vi "Apply.vi"(8 "error in (no error)":errorcluster, 11 "NEO480HTA Base CFG in":refnum<class "Read All CFG.lvclass">) -> (0 "error out":errorcluster, 3 "NEO480HTA Base CFG out":refnum<class "Read All CFG.lvclass">)   [LabVIEW 2023, in "NEO480HTA.lvlib" / "Read All CFG.lvclass"]
uses:
  Read All CFG.lvclass
  D:/git/HAL/HAL GOOP4/Configuration JSON Base/CFG JSON Base.lvclass
  Configuration JSON Base/CFG JSON Base.lvclass/CFG JSON Base.ctl
  Read All CFG.lvclass/Read All CFG.ctl
  9bca5c5c-edef-47c5-918c-bf756a254fce.vi
  fc27cf02-12b1-46f5-bd0d-6de24ae4e0a7.vi
  bc72a19a-b621-4a94-833b-c6b45453ec49.vi
  0be9cb3e-7191-46de-b2d2-d721f6475833.vi
  <vilib>/JDP Science/JSONtext/Find Item.vi
  <vilib>/JDP Science/JSONtext/Next JSON Value.vi
  <vilib>/JDP Science/JSONtext/String Subset.vi
  <vilib>/JDP Science/JSONtext/Parsing/Advance past next JSON Value (inlined COPY).vi
  <vilib>/JDP Science/JSONtext/Parsing/Advance past whitespace.vi
  <vilib>/JDP Science/JSONtext/Parsing/Advance past String.vi
  <vilib>/JDP Science/JSONtext/Parsing/Advance past Number.vi
  <vilib>/JDP Science/JSONtext/Parsing/Advance past Line Ending.vi
  <vilib>/JDP Science/JSONtext/Parsing/Parse Full Path or Item Name.vi
  <vilib>/JDP Science/JSONtext/Parsing/Advance past Array.vi
  <vilib>/JDP Science/JSONtext/Parsing/Advance past Object.vi
  <vilib>/JDP Science/JSONtext/support/Error Cluster From Code.vi
  <vilib>/JDP Science/JSONtext/Offset/Find Item Locations by Path.vi
  <vilib>/JDP Science/JSONtext/JSON text to Variant.vi
  <vilib>/Utility/error.llb/Error Cluster From Error Code.vi
  <vilib>/xnet/xnet.llb/XNET Create Session (Frame Input Single-point).vi
  <vilib>/JDP Science/JSONtext/LVClass Serializer/JSONtext LVClass Serializer.lvclass
  <vilib>/ErrorRing/Error Ring.xnode
  Configuration JSON Base/CFG JSON Base.lvclass
  <resource>/objmgr/xnet.rc
panel:
  out "Interface:CAN:Termination":u32(ring)=1 items=["Off", "On"]
  out "Timing Type":u32(ring)=1 items=["Cyclic Data", "Event Data", "Cyclic Remote", "Event Remote"]
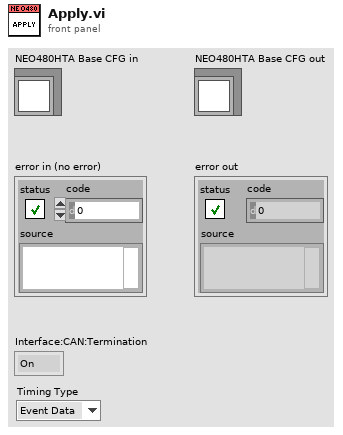
[diagram p1: front panel]
types:
  T1 = cluster{"Baud Rate":u32, "Comment":string, "Name":string}
  T2 = cluster{"Frame name":string, "Identifier":u32, "Payload Length":u32, "Timing Type":string, "Transmit Time":dbl, "Extended Identifier?":bool, "Comment":string}[]
  T3 = cluster{"Frame name":string, "Identifier":u32, "Payload Length":u32, "Timing Type":u32, "Transmit Time":dbl, "Extended Identifier?":bool, "Comment":string}
  T4 = typedef "LVStringsAndValuesArrayTypeDef_U32.ctl" = cluster{"String":string, "Value":u32}[]
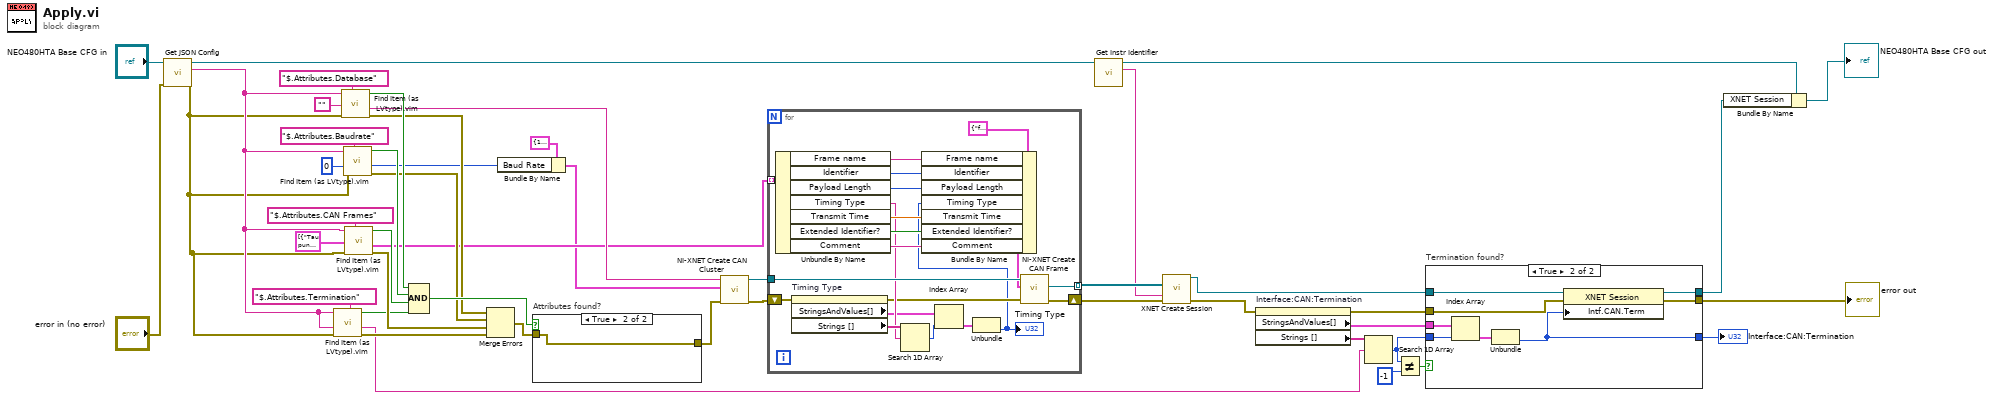
[diagram p0: block diagram]
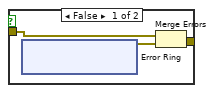
[diagram p3: hidden frame]
diagram:
  n1 = call "Get JSON Config.vi"("error in (no error)"="error in (no error)", "CFG Base in"="NEO480HTA Base CFG in") -> ("error out"=w7:errorcluster, "<JSON>Config>"=w8:string, "CFG Base out"=w29:refnum<class "Read All CFG.lvclass">)  [unwired: 7 in]
  n2 = call "Find Item (as LVtype).vim"("$Path or Item Name"="$.Attributes.Termination", "error in (no error)"=w7, "Data Type and Default Value"=w8, "JSON"=w8) -> ("error out"=w26:errorcluster, "Data"=w12:string, "Found"=w27:bool)  [unwired: 4 in, 1 out]
  n3 = call "Find Item (as LVtype).vim"("$Path or Item Name"="$.Attributes.Database", "error in (no error)"=w7, "Data Type and Default Value"="", "JSON"=w8) -> ("error out"=w33:errorcluster, "Data"=w40:string, "Found"=w41:bool)  [unwired: 4 in, 1 out]
  n4 = call "Find Item (as LVtype).vim"("$Path or Item Name"="$.Attributes.Baudrate", "error in (no error)"=w7, "Data Type and Default Value"=u32 0, "JSON"=w8) -> ("error out"=w34:errorcluster, "Data"=w20:u32, "Found"=w44:bool)  [unwired: 4 in, 1 out]
  n5 = call "Find Item (as LVtype).vim"("$Path or Item Name"="$.Attributes.CAN Frames", "error in (no error)"=w7, "Data Type and Default Value"=T2 [{"Frame name"="Taupunkt", "Identifier"=1152, "Payload Length"=8, "Timing Type"="Event Data", "Transmit Time"=0.0, "Extended Identifier?"=FALSE, "Comment"=""}], "JSON"=w8) -> ("error out"=w35:errorcluster, "Data"=w17:T2, "Found"=w45:bool)  [unwired: 4 in, 1 out]
  n6 = Compound Arithmetic op=AND(w41, w44, w45, w27) -> (w43:bool)
  n7 = Merge Errors(w33, w34, w35, w26) -> (w36:errorcluster)
  n8 = Bundle By Name(cluster=T1 {"Baud Rate"=125000, "Comment"="", "Name"="x"} ("CAN Cluster"), "Baud Rate"=w20) -> (w1:T1)
  n9 = case "Attributes found?" shown="True" w43 {
    tunnel: w36 -> [w49 w56]
    tunnel: [w50 w56] -> w39
    frame False {
      n10 = xnode "Error Ring"() -> ("error out"=w48:errorcluster)
      n11 = Merge Errors(w49, w48) -> (w50:errorcluster)
    }
    frame True {
    }
  }
  n12 = call "NI-XNET Create CAN Cluster.vi"("error in"=w39, "CAN Cluster"=w1, "database in"=w40) -> ("error out"=w37:errorcluster, "cluster out"=w38:refnum<k21>)  [unwired: 7 in]
  n13 = for {
    tunnel: w38 -> [w76]
    shift-right: [w75] -> w32
    shift-left: w37 -> [w64]
    tunnel: [w74] -> w18 mode=indexing
    tunnel: w17 -> [w73] mode=indexing
    n14 = Unbundle By Name(w73) -> ("Frame name"=w71:string, "Identifier"=w70:u32, "Payload Length"=w69:u32, "Timing Type"=w60:string, "Transmit Time"=w67:dbl, "Extended Identifier?"=w65:bool, "Comment"=w66:string)
    n15 = property on="Timing Type" class="Ring (strict)"(error in=w64) -> (error out=w58:errorcluster, "StringsAndValues[]"=w59:T4, "Strings []"=w61:string[])  [unwired: 1 in, 1 out]
    n16 = Search 1D Array(1D array=w61, element=w60) -> (index of element=w62:i32)  [unwired: 1 in]
    n17 = Index Array(array=w59, index=w62) -> (element=w63:cluster{"String":string, "Value":u32})
    n18 = Unbundle(w63) -> ("Value"=w57:u32)  [unwired: 1 out]
    "Timing Type" <- w57
    n19 = Bundle By Name(cluster=T3 {"Frame name"="frame1", "Identifier"=1, "Payload Length"=8, "Timing Type"=1, "Transmit Time"=0.0, "Extended Identifier?"=FALSE, "Comment"=""} ("CAN Frame"), "Frame name"=w71, "Identifier"=w70, "Payload Length"=w69, "Timing Type"=w57, "Transmit Time"=w67, "Extended Identifier?"=w65, "Comment"=w66) -> (w68:T3)
    n20 = call "NI-XNET Create CAN Frame.vi"("error in"=w58, "CAN Frame"=w68, "cluster in"=w76) -> ("error out"=w75:errorcluster, "frame out"=w74:refnum<k21>)  [unwired: 6 in, 1 out]
  }
  n21 = call-dynamic "Get Instr Identifier.vi"("Configuration Base in"=w29) -> ("Instr Identifier"=w9:string, "Configuration Base out"=w10:refnum<class "Read All CFG.lvclass">)  [unwired: 8 in, 1 out]
  n22 = call-poly <vilib>:"XNET Create Session.vi"("frame list"=w18, "interface"=w9, "error in (no error)"=w32) -> ("session out"=w25:refnum<k21>, "error out"=w14:errorcluster)  [unwired: 11 out]
  n23 = property on="Interface:CAN:Termination" class="Ring (strict)"(error in=w14) -> (error out=w13:errorcluster, "StringsAndValues[]"=w15:T4, "Strings []"=w16:string[])  [unwired: 1 in, 1 out]
  n24 = Search 1D Array(1D array=w16, element=w12) -> (index of element=w5:i32)  [unwired: 1 in]
  n25 = Not Equal?(x=w5, y=-1) -> (x != y?=w6:bool)
  n26 = case "Termination found?" shown="True" w6 {
    tunnel: w25 -> [w78 w87]
    tunnel: [w79 w86] -> w24
    tunnel: [w78 w85] -> w22
    tunnel: w5 -> [w77 w83]
    tunnel: w15 -> [_ w82]
    tunnel: w13 -> [w79 w81]
    tunnel: [w77 w80] -> w3
    frame False {
    }
    frame True {
      n27 = Index Array(array=w82, index=w83) -> (element=w84:cluster{"String":string, "Value":u32})
      n28 = Unbundle(w84) -> ("Value"=w80:u32)  [unwired: 1 out]
      n29 = property class="XNET Session"(reference=w87, error in=w81, "Intf.CAN.Term"=w80) -> (reference out=w85:refnum<k21>, error out=w86:errorcluster)
    }
  }
  "error out" <- w24
  "Interface:CAN:Termination" <- w3
  n30 = Bundle By Name(cluster=w10, "XNET Session"=w22) -> (→"NEO480HTA Base CFG out":refnum<class "Read All CFG.lvclass">)
